vi "create.TradeExpanded.vi"(8 "error in":errorcluster, 10 "TradeExpanded.Parameters":T1, 11 "TradeExpanded in":refnum<class "TradeExpanded.lvclass">) -> (0 "error out":errorcluster, 3 "TradeExpanded out":refnum<class "TradeExpanded.lvclass">)   [LabVIEW 2022 SP3, in "TradeExpanded.lvclass"]
uses:
  TradeExpanded.lvclass
  TradeExpanded.Parameters.ctl
  FieldSpec.ctl
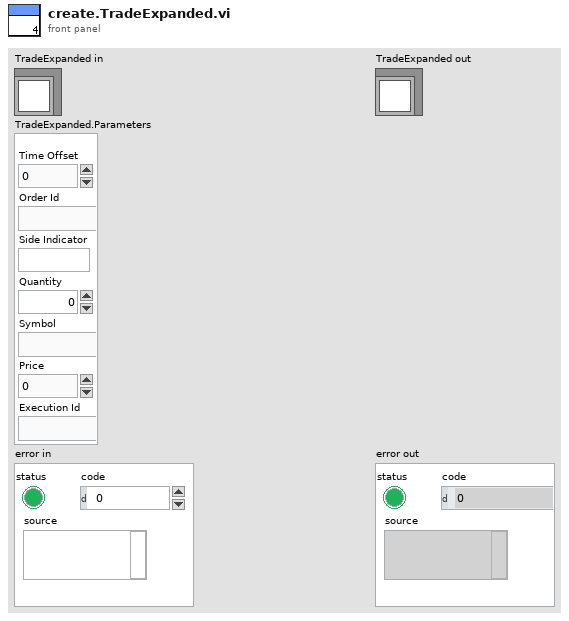
[diagram p1: front panel]
types:
  T1 = typedef "TradeExpanded.lvclass/TradeExpanded.Parameters.ctl" = cluster{"Time Offset":u32, "Order Id":string, "Side Indicator":string, "Quantity":u32, "Symbol":string, "Price":dbl, "Execution Id":string}
  T2 = typedef "FieldSpec.ctl" = cluster{"Name":string, "Offset":i32, "Length":i32, "FieldType":enum16{"Alphanumeric", "Binary", "BinaryLongPrice", "BinaryShortPrice", "BitField", "PrintableAscii", "Value"}, "FieldValue":variant}
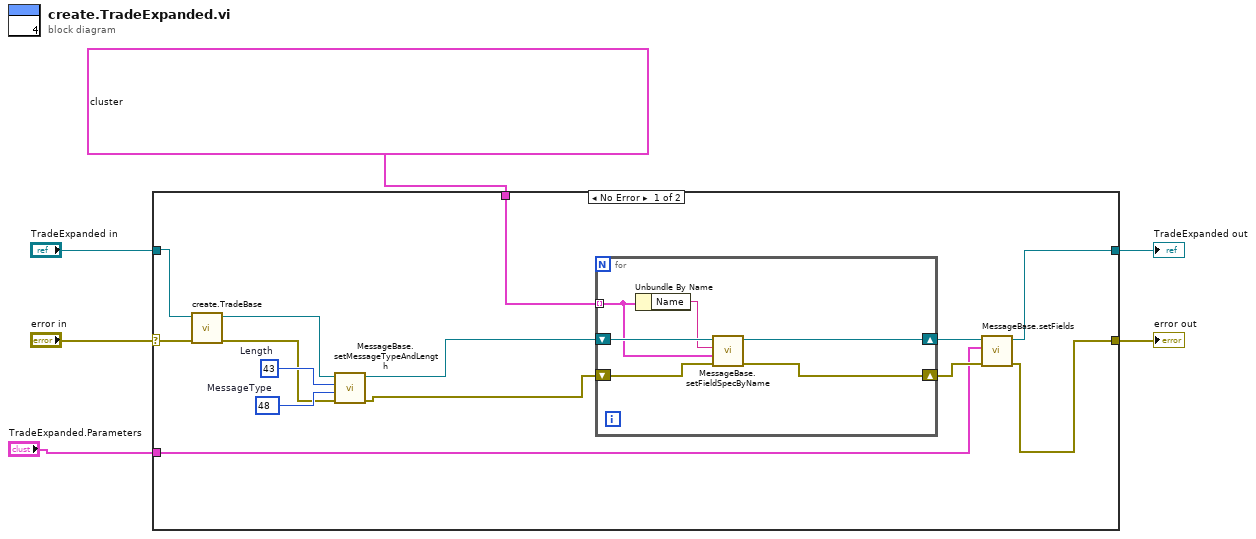
[diagram p0: block diagram]
diagram:
  n1 = case shown="No Error" "error in" {
    selector: "error in" -> [w15 w28]
    tunnel: [w9 w28] -> w5
    tunnel: [w8 w27] -> w3
    tunnel: "TradeExpanded in" -> [w16 w27]
    tunnel: "TradeExpanded.Parameters" -> [w12 _]
    tunnel: T2[] [{"Name"="Symbol", "Offset"=19, "Length"=8, "FieldType"=enum."PrintableAscii", "FieldValue"=variant}, {"Name"="Price", "Offset"=27, "Length"=8, "FieldType"=enum."BinaryLongPrice", "FieldValue"=variant}, {"Name"="Execution Id", "Offset"=35, "Length"=8, "FieldType"=enum."PrintableAscii", "FieldValue"=variant}] ("appended array") -> [w7 _]
    frame No Error {
      w19 = u8 48  # MessageType
      w20 = u8 43  # Length
      n2 = call-dynamic "create.TradeBase.vi"("error in (no error)"=w15, "TradeBase in"=w16) -> ("error out"=w18:errorcluster, "TradeBase out"=w17:refnum<class "TradeExpanded.lvclass">)  [unwired: 8 in]
      n3 = call-dynamic "MessageBase.setMessageTypeAndLength.vi"("error in (no error)"=w18, "MessageType"=w19, "Length"=w20, "MessageBase in"=w17) -> ("error out"=w11:errorcluster, "MessageBase out"=w10:refnum<class "TradeExpanded.lvclass">)  [unwired: 6 in]
      n4 = for {
        tunnel: w7 -> [w23] mode=indexing
        shift-right: [w22] -> w14
        shift-left: w10 -> [w26]
        shift-right: [w21] -> w13
        shift-left: w11 -> [w25]
        n5 = Unbundle By Name(w23) -> ("Name"=w24:string)
        n6 = call-dynamic "MessageBase.setFieldSpecByName.vi"("error in (no error)"=w25, "FIeldSpec"=w23, "Field.Name"=w24, "MessageBase in"=w26) -> ("error out"=w21:errorcluster, "MessageBase out"=w22:refnum<class "TradeExpanded.lvclass">)  [unwired: 6 in]
      }
      n7 = call-dynamic "MessageBase.setFields.vi"("error in (no error)"=w13, "Cluster (dup)"=w12, "MessageBase in"=w14) -> ("error out"=w9:errorcluster, "MessageBase out"=w8:refnum<class "TradeExpanded.lvclass">)  [unwired: 7 in]
    }
    frame Error {
    }
  }
  "error out" <- w5
  "TradeExpanded out" <- w3
